vi "FullAlign.vi"(0 "Joystick 0":dbl, 5 "Joystick 1":dbl, 7 "Distance":dbl=23.73829999999998, 9 "Angle":dbl=57.28800997198897, 11 "Button":bool=TRUE, 14 "Effort":dbl=0.2 format="%#_13g") -> (4 "Right Motor":dbl, 6 "Left Motor":dbl=-0.0, 8 "In Range?":bool, 13 "Sees Target?":bool=TRUE)   [LabVIEW 2016]
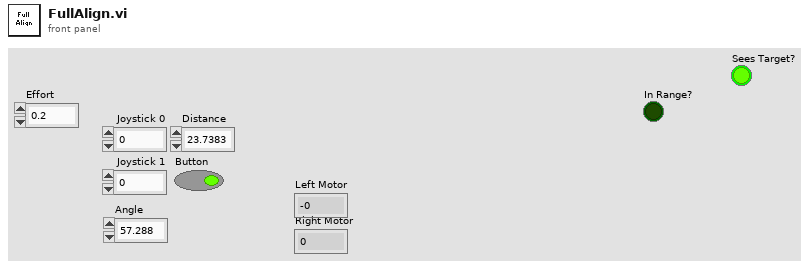
[diagram p1: front panel]
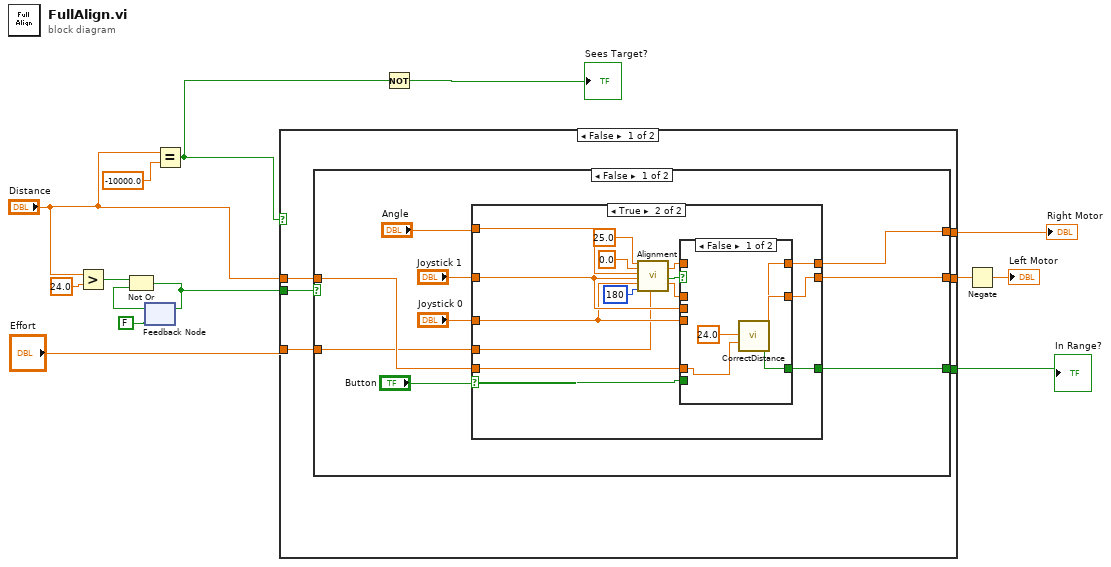
[diagram p0: block diagram]
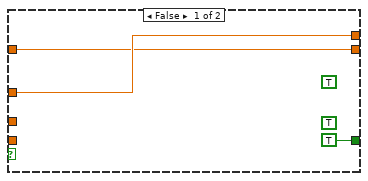
[diagram p2: hidden frame]
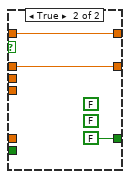
[diagram p3: hidden frame]
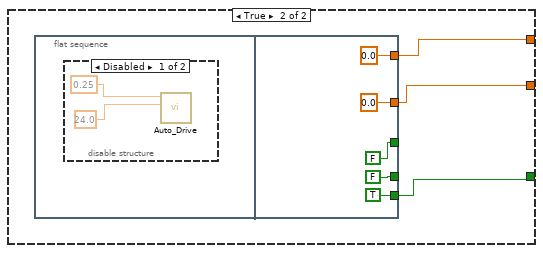
[diagram p4: hidden frame]
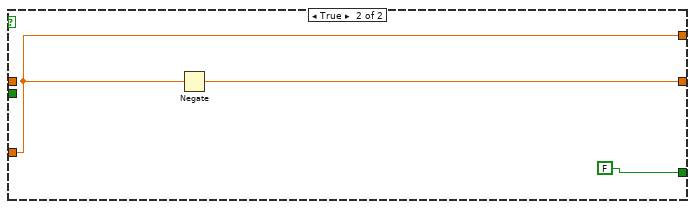
[diagram p6: hidden frame]
diagram:
  n1 = Greater?(x="Distance", y=24.0) -> (0:w11:bool)
  n2 = feedback #1(FALSE) -> (w12:bool)
  n3 = Not Or(1:w12, 2:w11) -> (0:w10:bool)
  n4 = feedback-in #1(w10) -> ()
  n5 = Equal?(x="Distance", y=-10000.0) -> (x = y?=w4:bool)
  n6 = case shown="False" w4 {
    tunnel: w10 -> [w20 _]
    tunnel: [w19 w67] -> w6
    tunnel: [w18 w66] -> w9
    tunnel: [w17 FALSE] -> w8
    tunnel: "Distance" -> [w16 _]
    tunnel: "Effort" -> [w15 w67]
    frame False {
      n7 = case shown="False" w20 {
        tunnel: w16 -> [w25 _]
        tunnel: [w24 w57] -> w19
        tunnel: [w23 w56] -> w18
        tunnel: [w22 w58] -> w17
        tunnel: w15 -> [w21 _]
        frame False {
          n8 = case shown="True" "Button" {
            selector: "Button" -> [_ w37]
            tunnel: "Joystick 1" -> [w31 w42]
            tunnel: "Joystick 0" -> [w32 w41]
            tunnel: [w31 w47] -> w23
            tunnel: [w32 w46] -> w24
            tunnel: "Angle" -> [_ w44]
            tunnel: [TRUE w36] -> w22
            tunnel: w25 -> [_ w35]
            tunnel: w21 -> [_ w33]
            frame False {
              (unwired) TRUE
              (unwired) TRUE
            }
            frame True {
              n9 = call "Alignment.vi"("Range"=25.0, "Target"=0.0, "Camera Feedback"=w44, "RightMotorSpeed"=w42, "LeftMotorSpeed"=w41, "POV"=180, "Turn_Gain"=w33) -> ("Right Motor"=w40:dbl, "LeftAndRight?"=w38:bool, "Left Motor"=w39:dbl)  [unwired: 10 in]
              n10 = case shown="False" w38 {
                tunnel: w42 -> [_ _]
                tunnel: w41 -> [_ _]
                tunnel: [w51 w54] -> w47
                tunnel: [w50 w55] -> w46
                tunnel: w37 -> [_ _]
                tunnel: w40 -> [_ w55]
                tunnel: w39 -> [_ w54]
                tunnel: [w48 FALSE] -> w36
                tunnel: w35 -> [w49 _]
                frame False {
                  n11 = call "CorrectDistance.vi"("CenterPoint"=24.0, "Distance"=w49) -> ("In Range?"=w48:bool, "Right Motor"=w50:dbl, "Left Motor"=w51:dbl)  [unwired: 23 in]
                }
                frame True {
                  (unwired) FALSE
                  (unwired) FALSE
                }
              }
            }
          }
        }
        frame True {
          n12 = flat-sequence {
            tunnel: [FALSE] -> _
            tunnel: [FALSE] -> _
            tunnel: [TRUE] -> w58
            tunnel: [0.0] -> w57
            tunnel: [0.0] -> w56
            frame #0 {
              n13 = disable-structure shown="Disabled" {
                frame Disabled {
                  n14 = call "Auto_Drive.vi"("distance"=24.0, "Drive Effort"=0.25) -> ()  [unwired: 10 in]
                }
                frame Enabled {
                }
              }
            }
            frame #1 {
            }
          }
        }
      }
    }
    frame True {
      n15 = Negate(x=w67) -> (-x=w66:dbl)
    }
  }
  "Right Motor" <- w6
  "In Range?" <- w8
  n16 = Not(x=w4) -> (.not. x?=→"Sees Target?":bool)
  n17 = Negate(x=w9) -> (-x=→"Left Motor":dbl)
